vi "Outline.vi"() -> ()   [LabVIEW 2019]
uses:
  <vilib>/PRIrvin/Graph Utilities/graph_utilities.lvclass/graph_utilities.ctl
  30be2593-79f7-4bd9-a4be-e507fb50de2d.vi
  <vilib>/PRIrvin/XY Utilities/subVIs/Subset (multiple).vi
  <vilib>/PRIrvin/XY Utilities/subVIs/Shift Zero (multiple).vi
  <vilib>/PRIrvin/XY Utilities/subVIs/Derivative (multiple).vi
  <vilib>/PRIrvin/XY Utilities/subVIs/Add float (multiple).vi
  <vilib>/PRIrvin/XY Utilities/subVIs/Subset (single).vi
  <vilib>/PRIrvin/XY Utilities/subVIs/Shift Zero (single).vi
  <vilib>/PRIrvin/XY Utilities/subVIs/Derivative (single).vi
  <vilib>/PRIrvin/XY Utilities/Swap X and Y.vi
  <vilib>/PRIrvin/XY Utilities/subVIs/Swap X and Y (single).vi
  <vilib>/Analysis/2dsp.llb/Derivative x(t).vi
  <vilib>/PRIrvin/XY Utilities/Private/X Array Index to Range.vi
  <vilib>/Utility/error.llb/Error Cluster From Error Code.vi
  <vilib>/gmath/interp.llb/Interpolate 1D.vi
  <userlib>/_MGI/1D Array/MGI Interpolate 1D Array Extended.vi
  <vilib>/Analysis/6fits.llb/Linear Fit.vi
  <vilib>/PRIrvin/Graph Utilities/XY Graph/Set XY Graph Value (array).vi
  <vilib>/PRIrvin/Graph Utilities/graph_utilities.lvclass
  <vilib>/PRIrvin/XY Utilities/xy_utilities.lvlib
  <userlib>/LevyLab/LV-Data/LV-Data/LV-Data.lvclass
  <userlib>/LevyLab/LV-Data/LV-Data.ITX/LV-Data.ITX.lvclass
panel:
  in  "parameter name":string="x data"
  in  "Write Path":path=path "C:/temp"
  in  "Read Path":path=path "C:/temp"
  in  "y data name":string="y data"
  in  "x data name":string="x data"
  out "XY Graph":cluster{"Intensity Data":dbl[], "Array":dbl[]}[](graph)
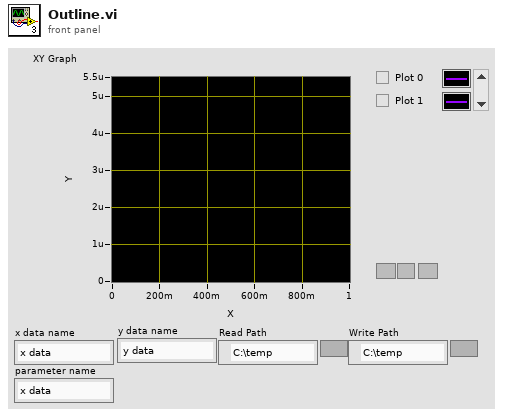
[diagram p1: front panel]
types:
  T1 = typedef "LV-Data.lvclass/Dictionary--cluster.ctl" = cluster{"key":string, "value":variant}
  T2 = typedef "Dictionary Object RefNum__ogtk.ctl" = refnum<k1>
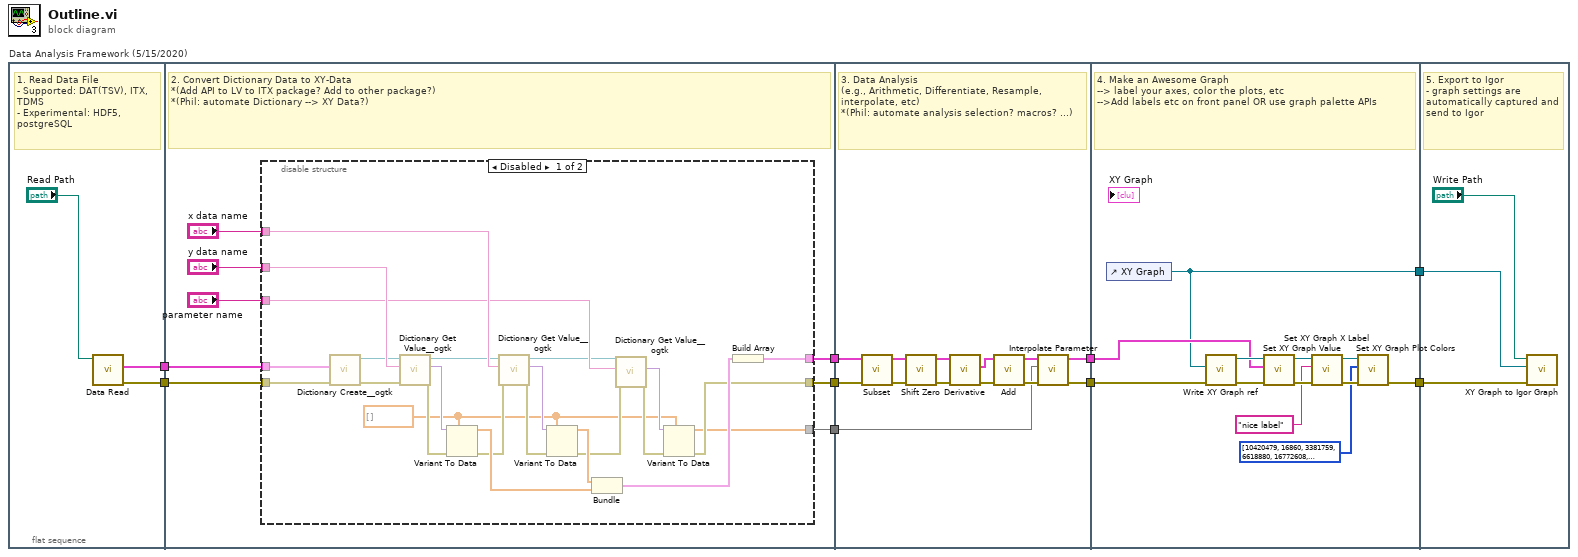
[diagram p0: block diagram]
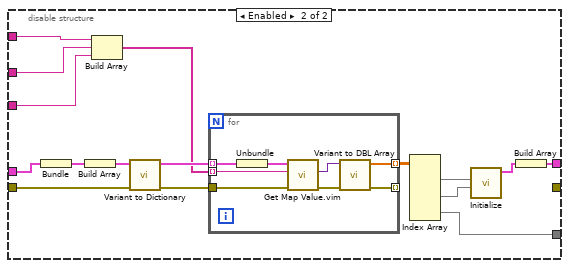
[diagram p2: hidden frame]
diagram:
  n1 = flat-sequence "Data Analysis Framework (5/15/2020)" {
    tunnel: [w11] -> w9
    tunnel: [w10] -> w8
    tunnel: w9 -> [w18]
    tunnel: w8 -> [w17]
    tunnel: [w16] -> w5
    tunnel: [w14] -> w2
    tunnel: [w13] -> w1
    tunnel: [w70] -> w7
    tunnel: w5 -> [w77]
    tunnel: [w71] -> w4
    tunnel: w2 -> [w76]
    tunnel: w1 -> [w69]
    tunnel: w7 -> [w90]
    tunnel: [w89] -> w6
    tunnel: w4 -> [w85]
    tunnel: [w84] -> w3
    tunnel: w6 -> [w95]
    tunnel: w3 -> [w94]
    frame #0 {
      # "1. Read Data File\n- Supported: DAT(TSV), ITX, TDMS\n- Experimental: HDF5, postgreSQL"
      n2 = call <userlib>:"Data Read.vi"("path"="Read Path") -> ("error out"=w11:errorcluster, "Data (Dictionary)"=w10:T1[])  [unwired: 7 in, 2 out]
    }
    frame #1 {
      # "2. Convert Dictionary Data to XY-Data\n*(Add API to LV to ITX package? Add to other package?)\n*(Phil: automate Dictionary --> XY Data?)"
      n3 = disable-structure shown="Disabled" {
        disable-tunnel: "x data name" -> [w44 w53]
        disable-tunnel: "y data name" -> [w36 w52]
        disable-tunnel: w18 -> [w32 w57]
        disable-tunnel: w17 -> [w31 w60]
        disable-tunnel: [w30 w48] -> w16
        disable-tunnel: "parameter name" -> [w27 w51]
        disable-tunnel: [w24 _] -> w14
        disable-tunnel: [w22 w45] -> w13
        frame Disabled {
          w23 = dbl[] []
          n4 = call <userlib>:"Dictionary Create__ogtk.vi"("error in (no error)"=w32, "initial dictionary (empty)"=w31) -> ("error out"=w33:errorcluster, "dictionary out"=w34:T2)  [unwired: 8 in]
          n5 = call <userlib>:"Dictionary Get Value__ogtk.vi"("error in"=w33, "key"=w36, "dictionary"=w34) -> ("error out"=w40:errorcluster, "value"=w37:variant, "dictionary out"=w35:T2)  [unwired: 5 in, 1 out]
          n6 = Variant To Data(error in=w40, type=w23, Variant=w37) -> (data=w42:dbl[], error out=w41:errorcluster)
          n7 = call <userlib>:"Dictionary Get Value__ogtk.vi"("error in"=w41, "key"=w44, "dictionary"=w35) -> ("error out"=w43:errorcluster, "value"=w38:variant, "dictionary out"=w21:T2)  [unwired: 5 in, 1 out]
          n8 = Variant To Data(error in=w43, type=w23, Variant=w38) -> (data=w39:dbl[], error out=w26:errorcluster)
          n9 = Bundle(w39, w42) -> (w29:cluster{dbl[], dbl[]})  [unwired: 1 in]
          n10 = call <userlib>:"Dictionary Get Value__ogtk.vi"("error in"=w26, "key"=w27, "dictionary"=w21) -> ("error out"=w25:errorcluster, "value"=w28:variant)  [unwired: 5 in, 2 out]
          n11 = Variant To Data(error in=w25, type=w23, Variant=w28) -> (data=w22:dbl[], error out=w24:errorcluster)
          n12 = Build Array(w29) -> (w30:cluster{dbl[], dbl[]}[])
        }
        frame Enabled {
          n13 = Bundle("Data (Dictionary)"=w60) -> (w59:cluster{"Data (Dictionary)":T1[]})  [unwired: 1 in]
          n14 = Build Array(w59) -> (w58:cluster{"Data (Dictionary)":T1[]}[])
          n15 = Build Array(w53, w52, w51) -> (w50:string[])
          n16 = call <userlib>:"Variant to Dictionary.vi"("error in (no error)"=w57, "Array in"=w58) -> ("error out"=w55:errorcluster, "Array out"=w56:cluster{"Data (Dictionary)":T1[]}[])  [unwired: 8 in]
          n17 = for {
            tunnel: [w66] -> _ mode=indexing
            tunnel: [w65] -> w54 mode=indexing
            tunnel: w56 -> [w64] mode=indexing
            tunnel: w55 -> [w62]
            tunnel: w50 -> [w61] mode=indexing
            n18 = Unbundle(w64) -> ("Data (Dictionary)"=w63:T1[])
            n19 = call "Get Map Value.vim"("error in (no error)"=w62, "Key"=w61, "map in"=w63) -> ("error out"=w67:errorcluster, "value"=w68:variant)  [unwired: 6 in, 1 out]
            n20 = call <userlib>:"Variant to DBL Array.vi"("error in (no error)"=w67, "Data (Variant)"=w68) -> ("error out"=w66:errorcluster, "1D Array"=w65:dbl[])  [unwired: 7 in, 1 out]
          }
          n21 = Index Array(array=w54) -> (element #1=w49:dbl[], element #2=w46:dbl[], element #3=w45:dbl[])  [unwired: 6 in]
          n22 = call <vilib>:"Initialize.vi"("Y-array"=w46, "X-array"=w49) -> ("XY-data out"=w47:cluster{"X-array":dbl[], "Y-array":dbl[]})  [unwired: 8 in, 1 out]
          n23 = Build Array(w47) -> (w48:cluster{"X-array":dbl[], "Y-array":dbl[]}[])
        }
      }
    }
    frame #2 {
      # "3. Data Analysis\n(e.g., Arithmetic, Differentiate, Resample, interpolate, etc)\n*(Phil: automate analysis selection? macros? ...)"
      n24 = call-poly <vilib>:"Subset.vi"("error in (no error)"=w76, "XY-data"=w77) -> ("error out"=w79:errorcluster, "Subset XY-data out"=w78:cluster{"X-array":dbl[], "Y-array":dbl[]}[])  [unwired: 8 in]
      n25 = call-poly <vilib>:"Shift Zero.vi"("error in (no error)"=w79, "XY-data"=w78) -> ("error out"=w74:errorcluster, "Shifted XY-data out"=w75:cluster{"X-array":dbl[], "Y-array":dbl[]}[])  [unwired: 8 in]
      n26 = call-poly <vilib>:"Derivative.vi"("error in (no error)"=w74, "XY-data"=w75) -> ("error out"=w80:errorcluster, "Differential out"=w81:cluster{"X-array":dbl[], "Y-array":dbl[]}[])  [unwired: 7 in, 1 out]
      n27 = call-poly <vilib>:"Add.vi"("error in (no error)"=w80, "XY-data"=w81) -> ("error out"=w73:errorcluster, "XY-data out"=w72:cluster{"X-array":dbl[], "Y-array":dbl[]}[])  [unwired: 8 in]
      n28 = call <vilib>:"Interpolate Parameter.vi"("error in (no error)"=w73, "Parameter-array"=w69, "XY-data"=w72) -> ("error out"=w70:errorcluster, "Interpolated XY-data out"=w71:cluster{"X-array":dbl[], "Y-array":dbl[]}[])  [unwired: 6 in, 1 out]
    }
    frame #3 {
      # "4. Make an Awesome Graph\n--> label your axes, color the plots, etc\n-->Add labels etc on front panel OR use graph palette APIs"
      n29 = control-ref of="XY Graph"() -> (w84:refnum<vi>)
      n30 = call <vilib>:"Write XY Graph ref.vi"("error in (no error)"=w90, "XY Graph"=w84) -> ("error out"=w88:errorcluster, "graph_utilities out"=w91:refnum<class "graph_utilities.lvclass">)  [unwired: 8 in]
      n31 = call-poly <vilib>:"Set XY Graph Value.vi"("error in (no error)"=w88, "XY-data"=w85, "graph_utilities in"=w91) -> ("error out"=w87:errorcluster, "graph_utilities out"=w92:refnum<class "graph_utilities.lvclass">)  [unwired: 7 in]
      n32 = call <vilib>:"Set XY Graph X Label.vi"("error in (no error)"=w87, "X Label"="nice label", "graph_utilities in"=w92) -> ("error out"=w86:errorcluster, "graph_utilities out"=w93:refnum<class "graph_utilities.lvclass">)  [unwired: 7 in]
      n33 = call <vilib>:"Set XY Graph Plot Colors.vi"("error in (no error)"=w86, "Colors []"=u32[] [10420479, 16860, 3381759, 6618880, 16772608, 16711680], "graph_utilities in"=w93) -> ("error out"=w89:errorcluster)  [unwired: 7 in, 1 out]
    }
    frame #4 {
      # "5. Export to Igor\n- graph settings are automatically captured and send to Igor"
      n34 = call <userlib>:"XY Graph to Igor Graph.vi"("error in (no error)"=w95, "XY Graph Reference"=w94, "Path"="Write Path") -> ()  [unwired: 7 in, 2 out]
    }
  }
